vi "averaged_ilemt_data.vi"(8 "error in":errorcluster, 9 "Position":dbl[](array[numeric]) format="%#_3p", 10 "Point time (ms)":u32=1, 11 "Settling time (ms)":u32=1) -> (0 "error out":errorcluster, 3 "Result string":string)   [LabVIEW 2014]
uses:
  ilemt_globals.vi
panel:
  # "Get ILEMT calibration log text output record, averaging over specified time"
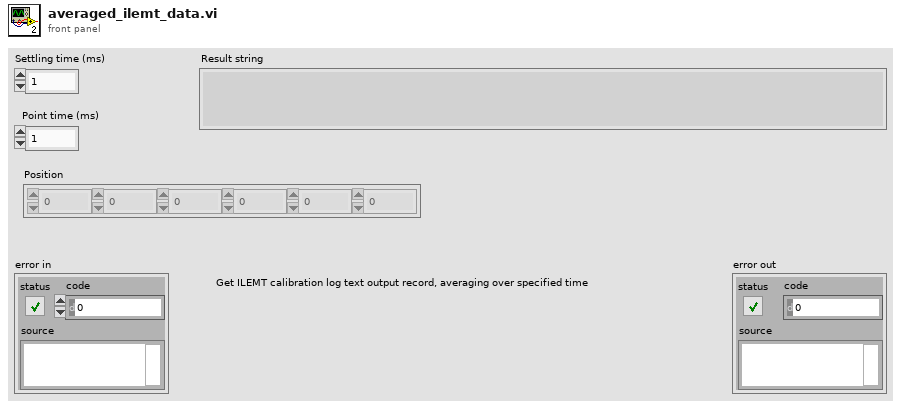
[diagram p1: front panel]
types:
  T1 = typedef "modulation_info.ctl" = cluster{"Fs full":dbl, "Fs high":dbl, "Fs low":dbl, "Read size":i32, "FFT size low":i32, "df low":dbl, "High carriers":dbl[], "Low carriers":dbl[], "Hi channels at low":i32[]}
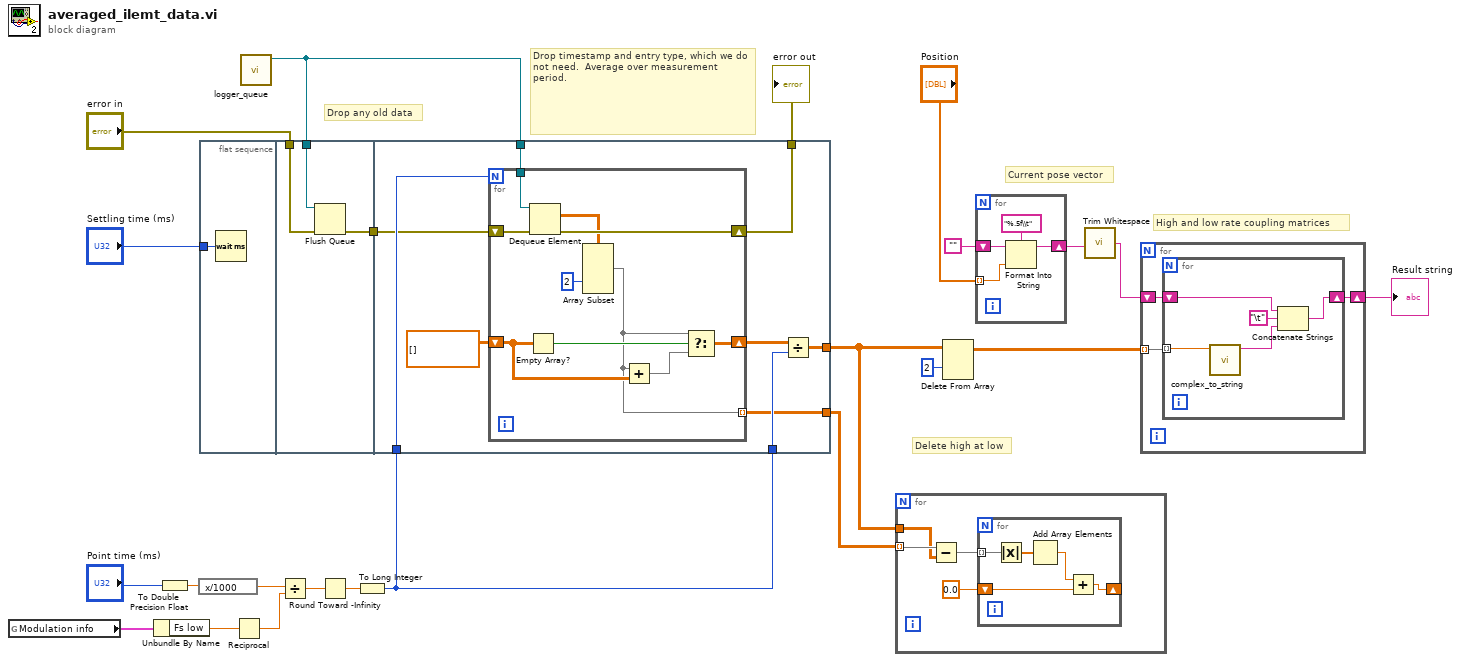
[diagram p0: block diagram]
diagram:
  # "Current pose vector"
  # "High and low rate coupling matrices"
  # "Delete high at low"
  # "Drop any old data"
  # "Drop timestamp and entry type, which we do not need.  Average over measurement period."
  n1 = global read "ilemt_globals.vi" "Modulation info"() -> (w22:T1)
  n2 = Unbundle By Name(w22) -> ("Fs low"=w21:dbl)
  n3 = To Double Precision Float(number="Point time (ms)") -> (double precision float=w20:dbl)
  n4 = expression code="x/1000"(w20) -> (w18:dbl)
  n5 = flat-sequence {
    tunnel: "Settling time (ms)" -> [w24]
    tunnel: w13 -> [w27]
    tunnel: "error in" -> [w26]
    tunnel: [w25] -> w11
    tunnel: w12 -> [w36]
    tunnel: w13 -> [w35]
    tunnel: w12 -> [w32]
    tunnel: w11 -> [w31]
    tunnel: [w30] -> w10
    tunnel: [w29] -> w2
    tunnel: [w28] -> w1
    frame #0 {
      n6 = Wait (ms)(milliseconds to wait=w24) -> ()  [unwired: 1 out]
    }
    frame #1 {
      n7 = Flush Queue(queue=w27, error in (no error)=w26) -> (error out=w25:errorcluster)  [unwired: 2 out]
    }
    frame #2 {
      n8 = for {
        N: w36 -> [_]
        tunnel: w35 -> [w46]
        shift-right: [w41] -> w33
        shift-left: cdb[][] [] -> [w40]
        shift-right: [w44] -> w30
        shift-left: w31 -> [w45]
        tunnel: [w37] -> w28 mode=indexing
        n9 = Empty Array?(array=w40) -> (empty?=w43:bool)
        n10 = Dequeue Element(queue=w46, error in (no error)=w45) -> (element=w39:cdb[][], error out=w44:errorcluster)  [unwired: 1 in, 2 out]
        n11 = Array Subset(array=w39, index (col)=2 ("index")) -> (w37:cdb[][])  [unwired: 3 in]
        n12 = Add(x=w37, y=w40) -> (x+y=w42:cdb[][])
        n13 = Select(t=w37, s=w43, f=w42) -> (s? t:f=w41:cdb[][])
      }
      n14 = Divide(x=w33, y=w32) -> (x/y=w29:cdb[][])
    }
  }
  n15 = Reciprocal(x=w21) -> (1/x=w17:dbl)
  n16 = call "logger_queue.vi"() -> ("queue out"=w13:refnum<queue>)  [unwired: 10 in, 1 out]
  n17 = Divide(x=w18, y=w17) -> (x/y=w16:dbl)
  n18 = Round Toward -Infinity(1:w16) -> (0:w15:dbl)
  n19 = To Long Integer(number=w15) -> (32bit integer=w12:i32)
  n20 = for {
    tunnel: w2 -> [w49]
    tunnel: w1 -> [w50] mode=indexing
    n21 = Subtract(x=w50, y=w49) -> (x-y=w47:cdb[][])
    n22 = for {
      shift-right: [w51] -> _
      shift-left: 0.0 -> [w54]
      tunnel: w47 -> [w53] mode=indexing
      n23 = Absolute Value(x=w53) -> (abs(x)=w52:dbl[])
      n24 = Add Array Elements(numeric array=w52) -> (sum=w55:dbl)
      n25 = Add(x=w55, y=w54) -> (x+y=w51:dbl)
    }
  }
  n26 = Delete From Array(array=w2, index (row)=2) -> (array with subset deleted=w8:cdb[][])  [unwired: 2 in, 1 out]
  n27 = for {
    tunnel: "Position" -> [w56] mode=indexing
    shift-right: [w57] -> w4
    shift-left: "" -> [w58]
    n28 = Format Into String(format string="%.5f\\t" ("format (%.3f)"), initial string=w58, w56) -> (resulting string=w57:string)  [unwired: 1 in, 1 out]
  }
  n29 = call <vilib>:"Trim Whitespace.vi"("string"=w4) -> ("trimmed string"=w3:string)  [unwired: 1 in]
  n30 = for {
    tunnel: w8 -> [w62] mode=indexing
    shift-right: [w60] -> w7
    shift-left: w3 -> [w61]
    n31 = for {
      tunnel: w62 -> [w67] mode=indexing
      shift-right: [w63] -> w60
      shift-left: w61 -> [w64]
      n32 = call "complex_to_string.vi"("Numeric"=w67) -> ("output string"=w66:string)  [unwired: 10 in]
      n33 = Concatenate Strings(w64, "\t" ("string"), w66) -> (w63:string)
    }
  }
  "Result string" <- w7
  "error out" <- w10
